vi "Cp-Cpk-SD-Mean-Variance-Calc.vi"(7 "Measurement-ID":i32[](array[numeric])=[0, 1, 2], 8 "error in (no error)":errorcluster, 9 "length":u32=4, 10 "Initialization Data":T1={"Measurement-ID"=[1, 2], "Measurement Names"=["a", "b"], "NominalValues"=[1.5, 2.3], "LSL"=[1.0, 1.8], "USL"=[2.0, 2.8], "LCL"=[1.0, 1.8], "UCL"=[2.0, 2.8]}, 11 "Reduced2DArray":dbl[][](array[numeric])) -> (0 "error out":errorcluster, 2 "Statistical Parameters":string[][](array[string]))   [LabVIEW 2019, in "Zen Analytics.lvlib" / "Zen Analytics.lvclass"]
uses:
  Zen Analytics.lvclass
  <vilib>/Analysis/NI_AALBase.lvlib
types:
  T1 = cluster{"Measurement-ID":i32[], "Measurement Names":string[], "NominalValues":dbl[], "LSL":dbl[], "USL":dbl[], "LCL":dbl[], "UCL":dbl[]}
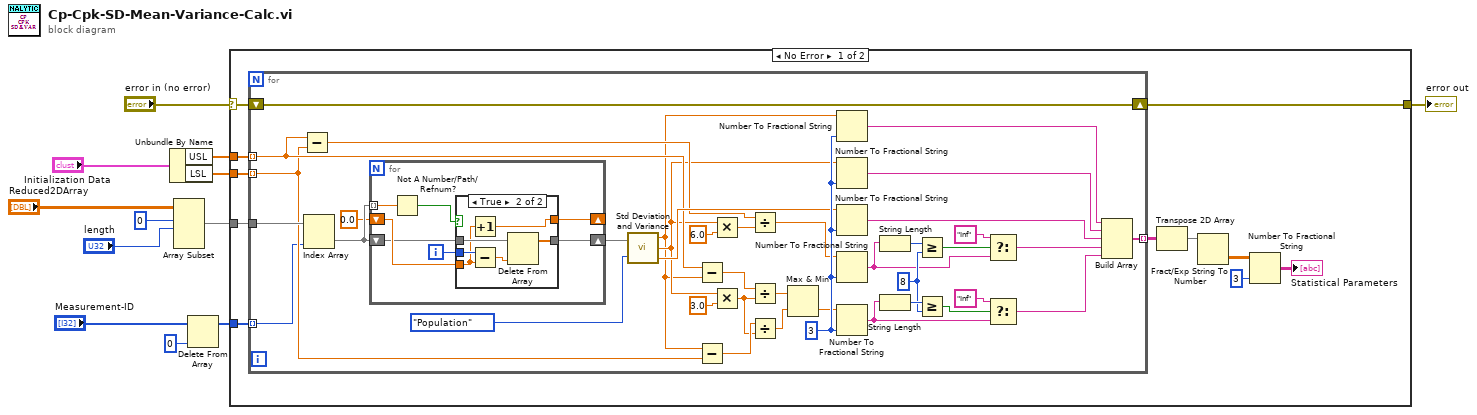
[diagram p0: block diagram]
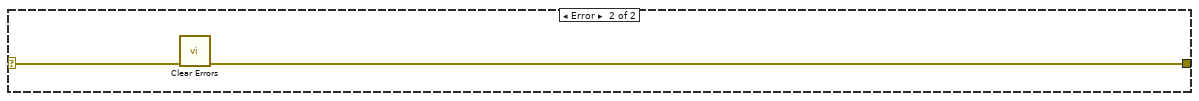
[diagram p3: hidden frame]
diagram:
  n1 = Unbundle By Name("Initialization Data") -> ("USL"=w6:dbl[], "LSL"=w5:dbl[])
  n2 = Array Subset(array="Reduced2DArray", index (row)=0 ("index"), length (row)="length") -> (w12:dbl[][])  [unwired: 2 in]
  n3 = Delete From Array(array="Measurement-ID", index=0) -> (array with subset deleted=w2:i32[])  [unwired: 1 in, 1 out]
  n4 = case shown="No Error" "error in (no error)" {
    selector: "error in (no error)" -> [w23 w79]
    tunnel: [w19 w78] -> w8
    tunnel: w12 -> [w22 _]
    tunnel: w6 -> [w21 _]
    tunnel: w5 -> [w20 _]
    tunnel: w2 -> [w14 _]
    frame No Error {
      n5 = for {
        tunnel: [w59] -> w18 mode=indexing
        tunnel: w22 -> [w58]
        tunnel: w21 -> [w49] mode=indexing
        tunnel: w20 -> [w45] mode=indexing
        tunnel: w14 -> [w28] mode=indexing
        shift-right: [w57] -> w19
        shift-left: w23 -> [w57]
        w31 = 8 ("y")
        w55 = i16 3 ("precision (6)")
        n6 = Subtract(x=w49, y=w45) -> (x-y=w53:dbl)
        n7 = Index Array(array=w58, index (col)=w28) -> (element=w27:dbl[])  [unwired: 1 in]
        n8 = for {
          tunnel: w27 -> [w69] mode=indexing
          shift-right: [w66] -> _
          shift-left: 0.0 -> [w67]
          shift-right: [w63] -> w26
          shift-left: w27 -> [w64]
          i -> [w65]
          n9 = Not A Number/Path/Refnum?(number/path/refnum=w69) -> (NaN/Path/Refnum?=w68:bool)
          n10 = case shown="True" w68 {
            tunnel: w64 -> [w70 w77]
            tunnel: w67 -> [w71 w72]
            tunnel: [w71 w75] -> w66
            tunnel: [w70 w76] -> w63
            tunnel: w65 -> [_ w73]
            frame False {
            }
            frame True {
              n11 = Increment(x=w72) -> (x+1=w75:dbl)
              n12 = Subtract(x=w73, y=w72) -> (x-y=w74:dbl)
              n13 = Delete From Array(array=w77, index=w74) -> (array with subset deleted=w76:dbl[])  [unwired: 1 in, 1 out]
            }
          }
        }
        n14 = call <vilib>:"Std Deviation and Variance.vi"("X"=w26, "Weighting (Sample)"=enum16{"Sample", "Population"}."Population") -> ("mean"=w24:dbl, "standard deviation"=w48:dbl, "variance"=w54:dbl)
        n15 = Subtract(x=w49, y=w24) -> (x-y=w46:dbl)
        n16 = Subtract(x=w24, y=w45) -> (x-y=w44:dbl)
        n17 = Multiply(x=w48, y=6.0) -> (x*y=w51:dbl)
        n18 = Multiply(x=w48, y=3.0) -> (x*y=w43:dbl)
        n19 = Divide(x=w53, y=w51) -> (x/y=w50:dbl)
        n20 = Divide(x=w46, y=w43) -> (x/y=w42:dbl)
        n21 = Divide(x=w44, y=w43) -> (x/y=w41:dbl)
        n22 = Max & Min(x=w42, y=w41) -> (min(x,y)=w40:dbl)  [unwired: 1 out]
        n23 = Number To Fractional String(number=w24, precision (6)=w55) -> (F-format string=w61:string)  [unwired: 2 in]
        n24 = Number To Fractional String(number=w48, precision (6)=w55) -> (F-format string=w60:string)  [unwired: 2 in]
        n25 = Number To Fractional String(number=w54, precision (6)=w55) -> (F-format string=w56:string)  [unwired: 2 in]
        n26 = Number To Fractional String(number=w50, precision (6)=w55) -> (F-format string=w30:string)  [unwired: 2 in]
        n27 = Number To Fractional String(number=w40, precision (6)=w55) -> (F-format string=w37:string)  [unwired: 2 in]
        n28 = String Length(string=w30) -> (length=w33:i32)
        n29 = String Length(string=w37) -> (length=w38:i32)
        n30 = Greater Or Equal?(x=w33, y=w31) -> (x >= y?=w32:bool)
        n31 = Greater Or Equal?(x=w38, y=w31) -> (x >= y?=w39:bool)
        n32 = Select(t="Inf", s=w32, f=w30) -> (s? t:f=w29:string)
        n33 = Select(t="Inf", s=w39, f=w37) -> (s? t:f=w35:string)
        n34 = Build Array(w61, w60, w56, w29, w35) -> (w59:string[])
      }
      n35 = Transpose 2D Array(2D array=w18) -> (transposed array=w17:string[][])
      n36 = Fract/Exp String To Number(string=w17) -> (number=w13:dbl[][])  [unwired: 3 in, 1 out]
      n37 = Number To Fractional String(number=w13, precision (6)=i16 3) -> (F-format string=→"Statistical Parameters":string[][])  [unwired: 2 in]
    }
    frame Error {
      n38 = call <vilib>:"Clear Errors.vi"("error in (no error)"=w79) -> ("error out"=w78:errorcluster)  [unwired: 5 in, 1 out]
    }
  }
  "error out" <- w8
